vi "DCS_Live_Plot.vi"() -> ()   [LabVIEW 2013]
uses:
  <vilib>/Utility/miscctls.llb/LVPointTypeDef.ctl
  <userlib>/_OpenG.lib/array/array.llb/Conditional Auto-Indexing Tunnel (DBL)__ogtk.vi
panel:
  out "DCS Array":dbl[][](array[numeric])
  in  "Changing?":bool
  in  "stop":bool
  in  "Tab Control":T1(tab)
  in  "Particle Limit":i32=1000
  out "Center Y":dbl
  out "Center X":dbl
  in  "Cursor Y":sgl min=-12 max=12 step=0.5
  in  "Cursor X":sgl min=-12 max=12 step=0.5
  in  "Select Position":T2(ring)
  in  "Distance from DCS 1":dbl min=-2.5 max=15.0 step=1.0 format="%.3f"
  in  "Distance from DCS 1 (m)":dbl(slide) scale=15.0..-2.5
  out "Live Plot":dbl[][](graph)
  in  "Min Time Stamp":timestamp
  out "Total No. of Particles":i32
  out "DCS 2 No. of Particles":i32
  out "DCS 1 No. of Particles":i32
  out "DCS 2":dbl[][](graph)
  out "DCS 1":dbl[][](graph)
  out "error out":errorcluster
  in  "error in (no error)":errorcluster
  # "DCS Live Plot"
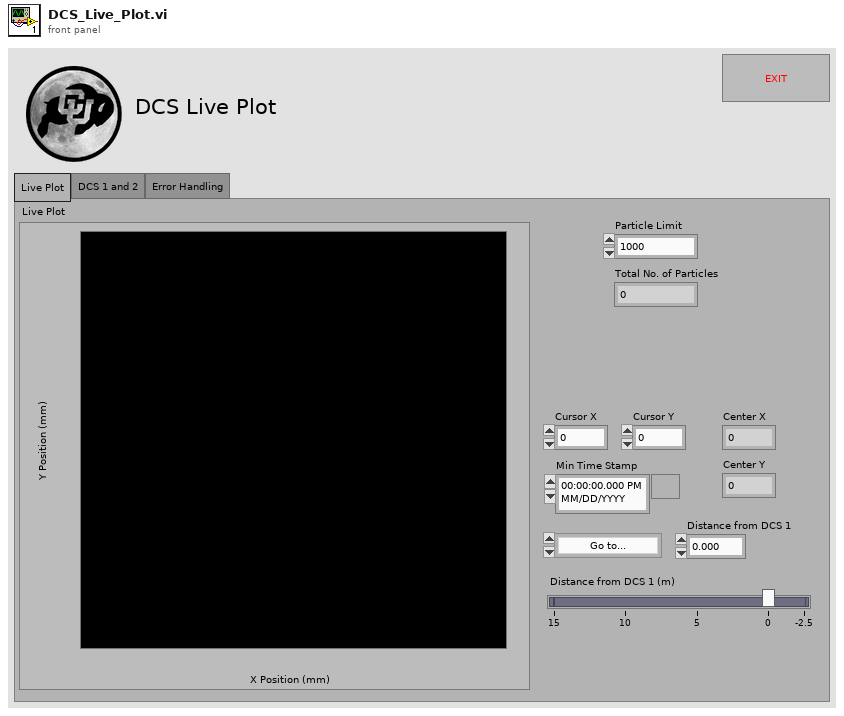
[diagram p1: front panel]
types:
  T1 = enum32{"Live Plot", "DCS 1 and 2", "Error Handling"}
  T2 = enum16{"Go to...", "DCS 1", "First Detector", "Second Detector", "PSU", "DCS 2", "Third Detector", "LEIL Front", "LEIL Center", "LEIL Back"}
  T3 = typedef "LVPointTypeDef.ctl" = cluster{"Horizontal":i16, "Vertical":i16}
  T4 = typedef "DisplayExperimentSetting.ctl" = cluster{"Current Experiment Name:":string, "Current Experiment Description:":string, "Current Experiment Group ID:":string, "Experiment Settings Last Updated At:":timestamp}
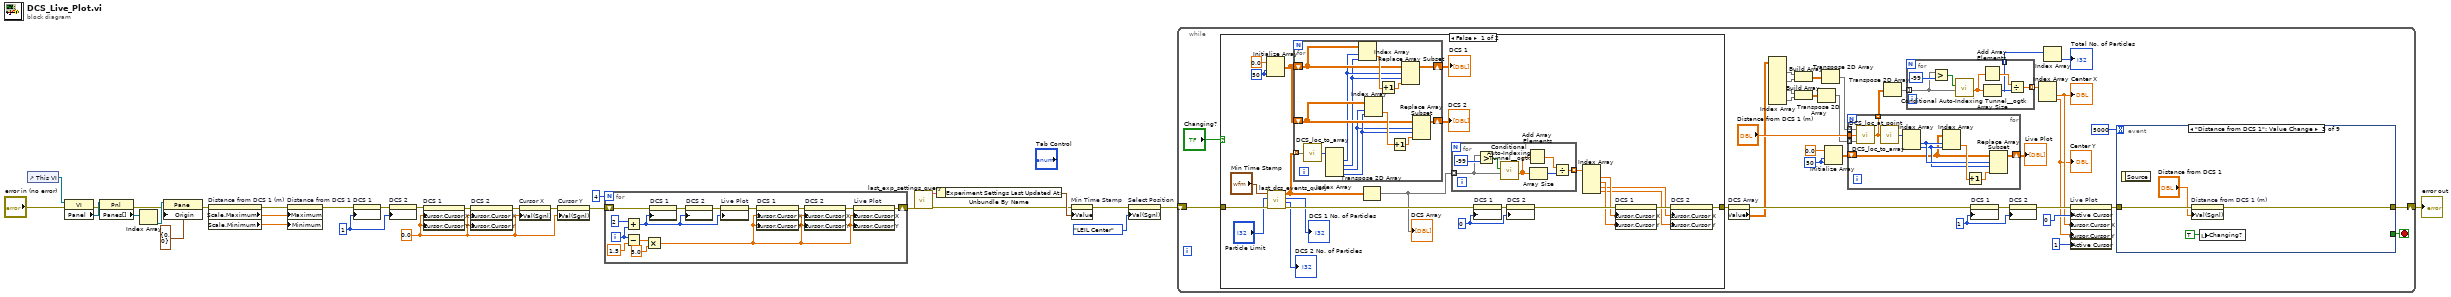
[diagram p0: block diagram]
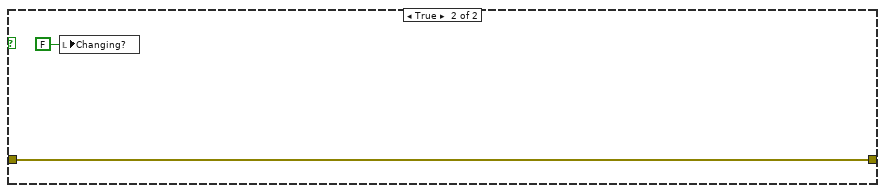
[diagram p2: hidden frame]
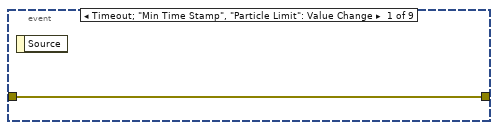
[diagram p3: hidden frame]
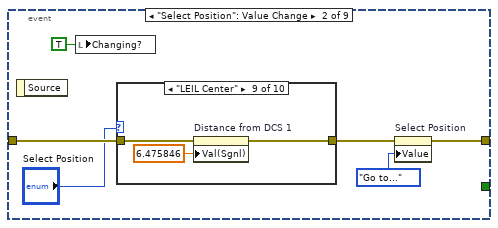
[diagram p4: hidden frame]
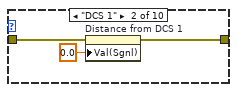
[diagram p6: hidden frame]
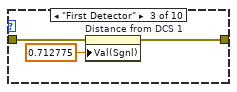
[diagram p7: hidden frame]
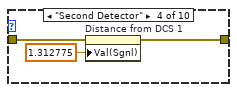
[diagram p8: hidden frame]
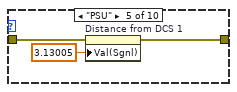
[diagram p9: hidden frame]
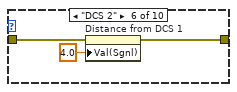
[diagram p10: hidden frame]
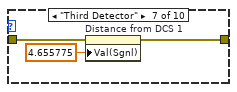
[diagram p11: hidden frame]
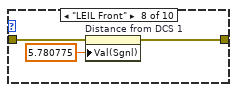
[diagram p12: hidden frame]
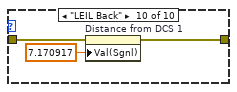
[diagram p13: hidden frame]
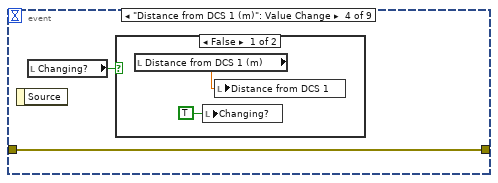
[diagram p14: hidden frame]
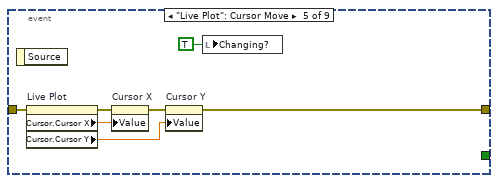
[diagram p16: hidden frame]
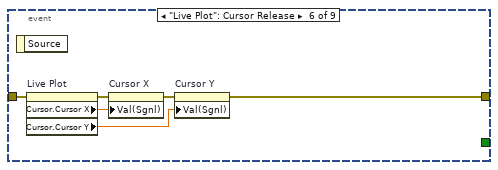
[diagram p17: hidden frame]
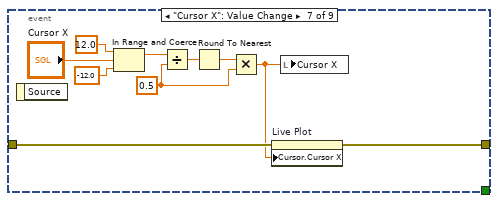
[diagram p18: hidden frame]
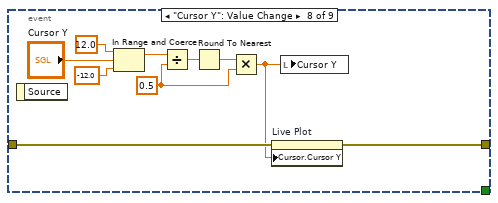
[diagram p19: hidden frame]
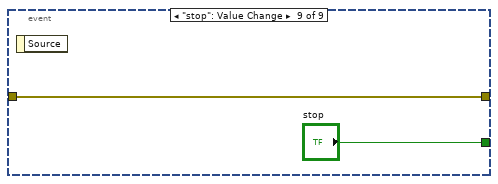
[diagram p20: hidden frame]
diagram:
  w8 = 0.0 ("Cursor.Cursor Position:Cursor X")
  w22 = u32 1 ("Active Cursor")
  n1 = control-ref of="This VI"() -> (w13:refnum<vi>)
  n2 = property class="VI"(reference=w13, error in="error in (no error)") -> (error out=w14:errorcluster, "Panel"=w15:refnum<vi>)  [unwired: 1 out]
  n3 = property class="Pnl"(reference=w15, error in=w14) -> (error out=w16:errorcluster, "Panes[]"=w17:refnum<vi>[])  [unwired: 1 out]
  n4 = Index Array(array=w17) -> (element=w18:refnum<vi>)  [unwired: 1 in]
  n5 = property class="Pane"(reference=w18, error in=w16, "Origin"=T3 {"Horizontal"=0, "Vertical"=0}) -> (error out=w5:errorcluster)  [unwired: 1 out]
  n6 = property on="Distance from DCS 1 (m)" class="Slide (strict)"(error in=w5) -> (error out=w2:errorcluster, "Scale.Maximum"=w4:dbl, "Scale.Minimum"=w3:dbl)  [unwired: 1 in, 1 out]
  n7 = property on="Distance from DCS 1" class="DigNum (strict)"(error in=w2, "Maximum"=w4, "Minimum"=w3) -> (error out=w1:errorcluster)  [unwired: 1 in, 1 out]
  n8 = property on="DCS 1" class="IntGraph (strict)"(error in=w1, "Active Cursor"=w22) -> (error out=w23:errorcluster)  [unwired: 1 in, 1 out]
  n9 = property on="DCS 2" class="IntGraph (strict)"(error in=w23, "Active Cursor"=w22) -> (error out=w6:errorcluster)  [unwired: 1 in, 1 out]
  n10 = property on="DCS 1" class="IntGraph (strict)"(error in=w6, "Cursor.Cursor X"=w8, "Cursor.Cursor Y"=w8) -> (error out=w24:errorcluster)  [unwired: 1 in, 1 out]
  n11 = property on="DCS 2" class="IntGraph (strict)"(error in=w24, "Cursor.Cursor X"=w8, "Cursor.Cursor Y"=w8) -> (error out=w10:errorcluster)  [unwired: 1 in, 1 out]
  n12 = property on="Cursor X" class="DigNum (strict)"(error in=w10, "Val(Sgnl)"=w8) -> (error out=w9:errorcluster)  [unwired: 1 in, 1 out]
  n13 = property on="Cursor Y" class="DigNum (strict)"(error in=w9, "Val(Sgnl)"=w8) -> (error out=w7:errorcluster)  [unwired: 1 in, 1 out]
  n14 = for {
    N: 4 -> [_]
    shift-right: [w35] -> w26
    shift-left: w7 -> [w42]
    i -> [w41]
    n15 = Add(x=2, y=w41) -> (x+y=w32:i32)
    n16 = Subtract(x=w41, y=1.5) -> (x-y=w39:dbl)
    n17 = Multiply(x=w39, y=5.0) -> (x*y=w34:dbl)
    n18 = property on="DCS 1" class="IntGraph (strict)"(error in=w42, "Active Cursor"=w32) -> (error out=w43:errorcluster)  [unwired: 1 in, 1 out]
    n19 = property on="DCS 2" class="IntGraph (strict)"(error in=w43, "Active Cursor"=w32) -> (error out=w33:errorcluster)  [unwired: 1 in, 1 out]
    n20 = property on="Live Plot" class="IntGraph (strict)"(error in=w33, "Active Cursor"=w32) -> (error out=w31:errorcluster)  [unwired: 1 in, 1 out]
    n21 = property on="DCS 1" class="IntGraph (strict)"(error in=w31, "Cursor.Cursor X"=w34, "Cursor.Cursor Y"=w34) -> (error out=w37:errorcluster)  [unwired: 1 in, 1 out]
    n22 = property on="DCS 2" class="IntGraph (strict)"(error in=w37, "Cursor.Cursor X"=w34, "Cursor.Cursor Y"=w34) -> (error out=w36:errorcluster)  [unwired: 1 in, 1 out]
    n23 = property on="Live Plot" class="IntGraph (strict)"(error in=w36, "Cursor.Cursor X"=w34, "Cursor.Cursor Y"=w34) -> (error out=w35:errorcluster)  [unwired: 1 in, 1 out]
  }
  n24 = call <userlib>:"last_exp_settings_query.vi"("error in (no error)"=w26) -> ("error out"=w27:errorcluster, "Experiment Settings"=w29:T4)  [unwired: 5 in, 4 out]
  n25 = Unbundle By Name(w29) -> ("Experiment Settings Last Updated At:"=w28:timestamp)
  n26 = property on="Min Time Stamp" class="AbsTime (strict)"(error in=w27, "Value"=w28) -> (error out=w11:errorcluster)  [unwired: 1 in, 1 out]
  n27 = property on="Select Position" class="Enum (strict)"(error in=w11, "Val(Sgnl)"=T2."LEIL Center" ("Select Position")) -> (error out=w21:errorcluster)  [unwired: 1 in, 1 out]
  n28 = while {
    shift-right: [w74] -> w30
    shift-left: w21 -> [w73]
    stop <- w78 stop-if-true
    w70 = 50 ("dimension size")
    w67 = u32 1 ("Active Cursor")
    n29 = case shown="False" "Changing?" {
      tunnel: w73 -> [w104 w131]
      tunnel: [w92 w131] -> w56
      frame False {
        w90 = u32 0 ("Active Cursor")
        w106 = 50 ("dimension size")
        n30 = Initialize Array(0.0 ("element"), w106, w106) -> (w103:dbl[][])
        n31 = call <userlib>:"last_dcs_events_query.vi"("error in (no error)"=w104, "Limit"="Particle Limit", "Min Time Stamp"="Min Time Stamp") -> ("error out"=w101:errorcluster, "No. of DCS 2 particles"=→"DCS 2 No. of Particles":i32, "No. of DCS 1 particles"=→"DCS 1 No. of Particles":i32, "DCS Array"=w91:dbl[][])  [unwired: 5 in]
        n32 = for {
          tunnel: w91 -> [w124] mode=indexing
          shift-right: [w123] -> w105
          shift-left: w103 -> [w122]
          shift-right: [w120] -> w102
          shift-left: w103 -> [w121]
          n33 = call <userlib>:"DCS_loc_to_array.vi"("DCS locs in"=w124) -> ("Array locs out"=w125:i32[])
          n34 = Index Array(array=w125) -> (element #1=w119:i32, element #2=w116:i32, element #3=w117:i32, element #4=w118:i32)  [unwired: 4 in]
          n35 = Index Array(array=w122, index (row)=w119, index (col)=w116) -> (element=w129:dbl)
          n36 = Index Array(array=w121, index (row)=w117, index (col)=w118) -> (element=w126:dbl)
          n37 = Increment(x=w129) -> (x+1=w128:dbl)
          n38 = Increment(x=w126) -> (x+1=w127:dbl)
          n39 = Replace Array Subset(array=w122, new element=w128, index (row)=w119, index (col)=w116) -> (w123:dbl[][])
          n40 = Replace Array Subset(array=w121, new element=w127, index (row)=w117, index (col)=w118) -> (w120:dbl[][])
        }
        "DCS 1" <- w105
        "DCS 2" <- w102
        n41 = Transpose 2D Array(2D array=w91) -> (transposed array=w86:dbl[][])
        "DCS Array" <- w86
        n42 = for {
          tunnel: [w113] -> w97 mode=indexing
          tunnel: w86 -> [w112] mode=indexing
          n43 = Greater?(x=w112, y=-99 ("Numeric")) -> (0:w111:bool[])
          n44 = call-poly <userlib>:"Conditional Auto-Indexing Tunnel__ogtk.vi"("Array in"=w112, "Elements to keep"=w111) -> ("Filtered Array out"=w110:dbl[])  [unwired: 5 in]
          n45 = Add Array Elements(numeric array=w110) -> (sum=w115:dbl)
          n46 = Array Size(array=w110) -> (size(s)=w109:i32)
          n47 = Divide(x=w115, y=w109) -> (x/y=w113:dbl)
        }
        n48 = property on="DCS 1" class="IntGraph (strict)"(error in=w101, "Active Cursor"=w90) -> (error out=w100:errorcluster)  [unwired: 1 in, 1 out]
        n49 = property on="DCS 2" class="IntGraph (strict)"(error in=w100, "Active Cursor"=w90) -> (error out=w98:errorcluster)  [unwired: 1 in, 1 out]
        n50 = Index Array(array=w97) -> (element #1=w96:dbl, element #2=w95:dbl, element #3=w94:dbl, element #4=w93:dbl)  [unwired: 4 in]
        n51 = property on="DCS 1" class="IntGraph (strict)"(error in=w98, "Cursor.Cursor X"=w96, "Cursor.Cursor Y"=w95) -> (error out=w99:errorcluster)  [unwired: 1 in, 1 out]
        n52 = property on="DCS 2" class="IntGraph (strict)"(error in=w99, "Cursor.Cursor X"=w94, "Cursor.Cursor Y"=w93) -> (error out=w92:errorcluster)  [unwired: 1 in, 1 out]
      }
      frame True {
        n53 = local write "Changing?"(FALSE ("Changing?")) -> ()
      }
    }
    n54 = property on="DCS Array" class="Arr (strict)"(error in=w56) -> (error out=w55:errorcluster, "Value"=w54:dbl[][])  [unwired: 1 in, 1 out]
    n55 = Index Array(array=w54) -> (element #1=w60:dbl[], element #2=w59:dbl[], element #3=w62:dbl[], element #4=w61:dbl[])  [unwired: 8 in]
    n56 = Build Array(w60, w59) -> (w58:dbl[][])
    n57 = Build Array(w62, w61) -> (w57:dbl[][])
    n58 = Transpose 2D Array(2D array=w57) -> (transposed array=w52:dbl[][])
    n59 = Transpose 2D Array(2D array=w58) -> (transposed array=w53:dbl[][])
    n60 = Initialize Array(0.0 ("element"), w70, w70) -> (w68:dbl[][])
    n61 = for {
      tunnel: w53 -> [w140] mode=indexing
      tunnel: w52 -> [w139] mode=indexing
      tunnel: "Distance from DCS 1 (m)" -> [w138]
      shift-right: [w135] -> w71
      shift-left: w68 -> [w134]
      tunnel: [w132] -> w51 mode=indexing
      n62 = call <userlib>:"DCS_loc_at_point.vi"("DCS 2 Loc"=w139, "Distance from DCS 1"=w138, "DCS 1 Loc"=w140) -> ("Current Loc"=w132:dbl[])
      n63 = call <userlib>:"DCS_loc_to_array.vi"("DCS locs in"=w132) -> ("Array locs out"=w133:i32[])
      n64 = Index Array(array=w133) -> (element #1=w137:i32, element #2=w136:i32)  [unwired: 2 in]
      n65 = Index Array(array=w134, index (row)=w137, index (col)=w136) -> (element=w142:dbl)
      n66 = Increment(x=w142) -> (x+1=w141:dbl)
      n67 = Replace Array Subset(array=w134, new element=w141, index (row)=w137, index (col)=w136) -> (w135:dbl[][])
    }
    "Live Plot" <- w71
    n68 = Transpose 2D Array(2D array=w51) -> (transposed array=w50:dbl[][])
    n69 = for {
      tunnel: [w82] -> w66 mode=indexing
      tunnel: w50 -> [w81] mode=indexing
      tunnel: [w79] -> w45 mode=indexing
      n70 = Greater?(x=w81, y=-99 ("Numeric")) -> (0:w80:bool[])
      n71 = call-poly <userlib>:"Conditional Auto-Indexing Tunnel__ogtk.vi"("Array in"=w81, "Elements to keep"=w80) -> ("Filtered Array out"=w83:dbl[])  [unwired: 5 in]
      n72 = Add Array Elements(numeric array=w83) -> (sum=w85:dbl)
      n73 = Array Size(array=w83) -> (size(s)=w79:i32)
      n74 = Divide(x=w85, y=w79) -> (x/y=w82:dbl)
    }
    n75 = property on="DCS 1" class="IntGraph (strict)"(error in=w55, "Active Cursor"=w67) -> (error out=w76:errorcluster)  [unwired: 1 in, 1 out]
    n76 = property on="DCS 2" class="IntGraph (strict)"(error in=w76, "Active Cursor"=w67) -> (error out=w65:errorcluster)  [unwired: 1 in, 1 out]
    n77 = Index Array(array=w66) -> (element #1=w48:dbl, element #2=w47:dbl)  [unwired: 2 in]
    "Center X" <- w48
    "Center Y" <- w47
    n78 = Index Array(array=w45) -> (element=→"Total No. of Particles":i32)  [unwired: 1 in]
    n79 = property on="Live Plot" class="IntGraph (strict)"(error in=w65, "Active Cursor"=u32 0, "Cursor.Cursor X"=w48, "Cursor.Cursor Y"=w47, "Active Cursor"=u32 1) -> (error out=w49:errorcluster)  [unwired: 1 in, 1 out]
    n80 = event shown="[2] \"Distance from DCS 1\": Value Change" {
      selector: _ -> [_ _ _ _ _ _ _ _ _]
      dyn-events: _ -> [_ _ _ _ _ _ _ _ _]
      timeout: 5000 -> [_ _ _ _ _ _ _ _ _]
      tunnel: [_ _ _ _ _ _ _ _ "stop"] -> w78
      tunnel: w49 -> [w143 w149 w181 w183 w192 w198 w208 w218 w219]
      tunnel: [w143 w146 w180 w183 w187 w193 w207 w217 w219] -> w74
      event Timeout; "Min Time Stamp", "Particle Limit": Value Change {
        n81 = event-data() -> ()  [unwired: 1 in, 1 out]
      }
      event "Select Position": Value Change {
        n82 = event-data() -> ()  [unwired: 1 in, 1 out]
        n83 = local write "Changing?"(TRUE ("Changing?")) -> ()
        n84 = case shown="\"LEIL Center\"" "Select Position" {
          tunnel: w149 -> [w150 w153 w156 w159 w162 w165 w168 w171 w174 w177]
          tunnel: [w150 w152 w155 w158 w161 w164 w167 w170 w173 w176] -> w147
          frame "Go to..." {
          }
          frame "DCS 1" {
            n85 = property on="Distance from DCS 1" class="DigNum (strict)"(error in=w153, "Val(Sgnl)"=0.0 ("Value (Signaling)")) -> (error out=w152:errorcluster)  [unwired: 1 in, 1 out]
          }
          frame "First Detector" {
            n86 = property on="Distance from DCS 1" class="DigNum (strict)"(error in=w156, "Val(Sgnl)"=0.712775 ("Value (Signaling)")) -> (error out=w155:errorcluster)  [unwired: 1 in, 1 out]
          }
          frame "Second Detector" {
            n87 = property on="Distance from DCS 1" class="DigNum (strict)"(error in=w159, "Val(Sgnl)"=1.312775 ("Value (Signaling)")) -> (error out=w158:errorcluster)  [unwired: 1 in, 1 out]
          }
          frame "PSU" {
            n88 = property on="Distance from DCS 1" class="DigNum (strict)"(error in=w162, "Val(Sgnl)"=3.13005 ("Value (Signaling)")) -> (error out=w161:errorcluster)  [unwired: 1 in, 1 out]
          }
          frame "DCS 2" {
            n89 = property on="Distance from DCS 1" class="DigNum (strict)"(error in=w165, "Val(Sgnl)"=4.0 ("Value (Signaling)")) -> (error out=w164:errorcluster)  [unwired: 1 in, 1 out]
          }
          frame "Third Detector" {
            n90 = property on="Distance from DCS 1" class="DigNum (strict)"(error in=w168, "Val(Sgnl)"=4.655775 ("Value (Signaling)")) -> (error out=w167:errorcluster)  [unwired: 1 in, 1 out]
          }
          frame "LEIL Front" {
            n91 = property on="Distance from DCS 1" class="DigNum (strict)"(error in=w171, "Val(Sgnl)"=5.780775 ("Value (Signaling)")) -> (error out=w170:errorcluster)  [unwired: 1 in, 1 out]
          }
          frame "LEIL Center" {
            n92 = property on="Distance from DCS 1" class="DigNum (strict)"(error in=w174, "Val(Sgnl)"=6.475846 ("Value (Signaling)")) -> (error out=w173:errorcluster)  [unwired: 1 in, 1 out]
          }
          frame "LEIL Back" {
            n93 = property on="Distance from DCS 1" class="DigNum (strict)"(error in=w177, "Val(Sgnl)"=7.170917 ("Value (Signaling)")) -> (error out=w176:errorcluster)  [unwired: 1 in, 1 out]
          }
        }
        n94 = property on="Select Position" class="Enum (strict)"(error in=w147, "Value"=T2."Go to..." ("Select Position")) -> (error out=w146:errorcluster)  [unwired: 1 in, 1 out]
      }
      event "Distance from DCS 1": Value Change {
        n95 = event-data() -> ()  [unwired: 1 in, 1 out]
        n96 = property on="Distance from DCS 1 (m)" class="Slide (strict)"(error in=w181, "Val(Sgnl)"="Distance from DCS 1") -> (error out=w180:errorcluster)  [unwired: 1 in, 1 out]
        n97 = local write "Changing?"(TRUE ("Changing?")) -> ()
      }
      event "Distance from DCS 1 (m)": Value Change {
        n98 = event-data() -> ()  [unwired: 1 in, 1 out]
        n99 = local read "Changing?"() -> (w182:bool)
        n100 = case shown="False" w182 {
          frame False {
            n101 = local read "Distance from DCS 1 (m)"() -> (w185:dbl)
            n102 = local write "Changing?"(TRUE ("Changing?")) -> ()
            n103 = local write "Distance from DCS 1"(w185) -> ()
          }
          frame True {
          }
        }
      }
      event "Live Plot": Cursor Move {
        n104 = event-data() -> ()  [unwired: 1 in, 1 out]
        n105 = property on="Live Plot" class="IntGraph (strict)"(error in=w192) -> (error out=w191:errorcluster, "Cursor.Cursor X"=w190:dbl, "Cursor.Cursor Y"=w188:dbl)  [unwired: 1 in, 1 out]
        n106 = property on="Cursor X" class="DigNum (strict)"(error in=w191, "Value"=w190) -> (error out=w189:errorcluster)  [unwired: 1 in, 1 out]
        n107 = property on="Cursor Y" class="DigNum (strict)"(error in=w189, "Value"=w188) -> (error out=w187:errorcluster)  [unwired: 1 in, 1 out]
        n108 = local write "Changing?"(TRUE ("Changing?")) -> ()
      }
      event "Live Plot": Cursor Release {
        n109 = event-data() -> ()  [unwired: 1 in, 1 out]
        n110 = property on="Live Plot" class="IntGraph (strict)"(error in=w198) -> (error out=w197:errorcluster, "Cursor.Cursor X"=w196:dbl, "Cursor.Cursor Y"=w194:dbl)  [unwired: 1 in, 1 out]
        n111 = property on="Cursor X" class="DigNum (strict)"(error in=w197, "Val(Sgnl)"=w196) -> (error out=w195:errorcluster)  [unwired: 1 in, 1 out]
        n112 = property on="Cursor Y" class="DigNum (strict)"(error in=w195, "Val(Sgnl)"=w194) -> (error out=w193:errorcluster)  [unwired: 1 in, 1 out]
      }
      event "Cursor X": Value Change {
        w201 = sgl 0.5 ("y")
        n113 = event-data() -> ()  [unwired: 1 in, 1 out]
        n114 = In Range and Coerce(upper limit=sgl 12.0, x="Cursor X", lower limit=sgl -12.0) -> (coerced(x)=w204:sgl)  [unwired: 1 out]
        n115 = Divide(x=w204, y=w201) -> (x/y=w203:sgl)
        n116 = Round To Nearest(number=w203) -> (nearest integer value=w202:sgl)
        n117 = Multiply(x=w202, y=w201) -> (x*y=w199:sgl)
        n118 = property on="Live Plot" class="IntGraph (strict)"(error in=w208, "Cursor.Cursor X"=w199) -> (error out=w207:errorcluster)  [unwired: 1 in, 1 out]
        n119 = local write "Cursor X"(w199) -> ()
      }
      event "Cursor Y": Value Change {
        w211 = sgl 0.5 ("y")
        n120 = event-data() -> ()  [unwired: 1 in, 1 out]
        n121 = In Range and Coerce(upper limit=sgl 12.0, x="Cursor Y", lower limit=sgl -12.0) -> (coerced(x)=w214:sgl)  [unwired: 1 out]
        n122 = Divide(x=w214, y=w211) -> (x/y=w213:sgl)
        n123 = Round To Nearest(number=w213) -> (nearest integer value=w212:sgl)
        n124 = Multiply(x=w212, y=w211) -> (x*y=w209:sgl)
        n125 = property on="Live Plot" class="IntGraph (strict)"(error in=w218, "Cursor.Cursor Y"=w209) -> (error out=w217:errorcluster)  [unwired: 1 in, 1 out]
        n126 = local write "Cursor Y"(w209) -> ()
      }
      event "stop": Value Change {
        n127 = event-data() -> ()  [unwired: 1 in, 1 out]
      }
    }
  }
  "error out" <- w30
